vi "DatabaseHand_Create.vi"(8 "error in (no error)":errorcluster, 11 "Name":string) -> (0 "error out":errorcluster, 1 "Created New":bool, 3 "Database RefNum out":T1)   [LabVIEW 2016]
doc: "This VI finds the RefNum of an existing object with the input Name or creates a new object if the Name is not found or Name is unwired or an empty string.\nCopyright 2001 VI Engineering, Inc."
uses:
  private/vis/DatabaseHand_RefNum.ctl
  private/vis/DatabaseHand_Function.ctl
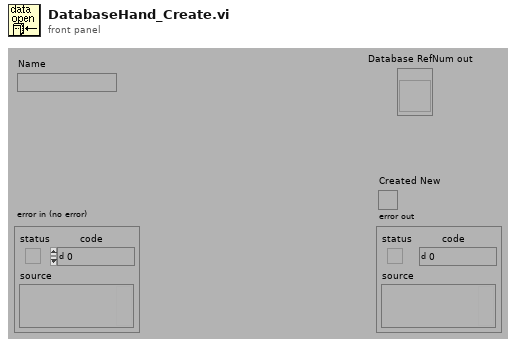
[diagram p1: front panel]
types:
  T1 = typedef "DatabaseHand_RefNum.ctl" = refnum<vi>
  T2 = typedef "DatabaseHand_Function.ctl" = enum16{"Reset", "Register", "Get Data", "Set Data", "Unregister", "Test", "Get Objects", "Delete Data"}
  T3 = typedef "Database_Refnum.ctl" = refnum<vi>
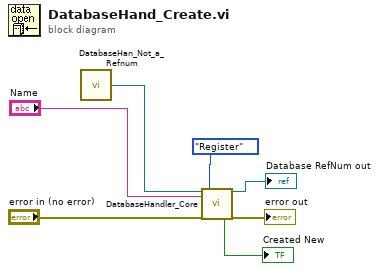
[diagram p0: block diagram]
diagram:
  n1 = call "DatabaseHan_Not_a_Refnum.vi"() -> ("Not_an_element_Refnum"=w2:T3)
  n2 = call "DatabaseHandler_Core.vi"("Object Refnum In"=w2, "Name"="Name", "error in (no error)"="error in (no error)", "Function (Get Data)"=DatabaseHand_Function."Register") -> ("Created New"=→"Created New":bool, "Object Refnum out"=→"Database RefNum out":T3, "error out"=→"error out":errorcluster)  [unwired: 3 in, 10 out]
